vi "Write PLC Config.vi"(8 "error in (no error)":errorcluster, 10 "PLC Config":T1={"Use TCP"=FALSE, "Reference Format"=6, "Swap Words"=FALSE, "Poll List"=[]} {"Reference Format" items=["4 Digits"=4, "5 Digits"=5, "6 Digits"=6]}, 11 "Modicon PLC in":refnum<class "MB PLC Client.lvclass">) -> (0 "error out":errorcluster, 3 "Modicon PLC out":refnum<class "MB PLC Client.lvclass">)   [LabVIEW 2018, in "MB PLC Client.lvlib" / "MB PLC Client.lvclass"]
uses:
  MB PLC Client.lvclass
  Types/PLC Config_Cluster.ctl
  Types/MB Ref Range_Cluster.ctl
  MB PLC Client.lvclass/MB PLC Client.ctl
  MB PLC Client.lvlib
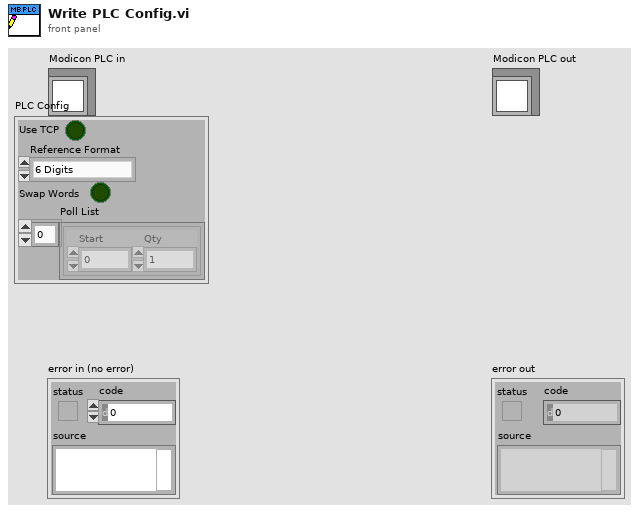
[diagram p1: front panel]
types:
  T1 = typedef "MB PLC Client.lvlib/PLC Config_Cluster.ctl" = cluster{"Use TCP":bool, "Reference Format":u16, "Swap Words":bool, "Poll List":T2[]}
  T2 = typedef "MB PLC Client.lvlib/MB Ref Range_Cluster.ctl" = cluster{"Start":u32, "Qty":u16}
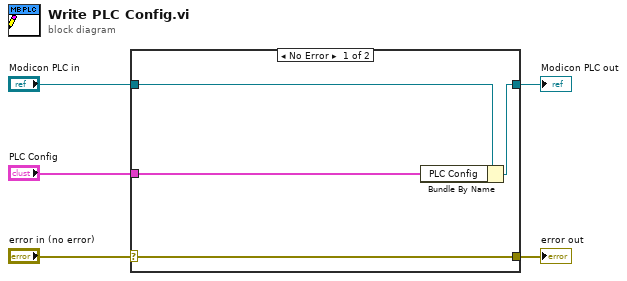
[diagram p0: block diagram]
diagram:
  n1 = case shown="No Error" "error in (no error)" {
    selector: "error in (no error)" -> [w9 w10]
    tunnel: [w9 w10] -> w4
    tunnel: [w7 w11] -> w2
    tunnel: "Modicon PLC in" -> [w8 w11]
    tunnel: "PLC Config" -> [w6 _]
    frame No Error {
      n2 = Bundle By Name(cluster=w8, "PLC Config"=w6) -> (w7:refnum<class "MB PLC Client.lvclass">)
    }
    frame Error {
    }
  }
  "error out" <- w4
  "Modicon PLC out" <- w2
